vi "ReversedEngineering AnalyseStateMachineWhileLoop.vi"(0 "OutSideWhileLoop":refnum<vi>, 1 "StateWhileLoop":refnum<vi>, 2 "SelStrings":string[](array[string]), 5 "error in":errorcluster) -> (15 "InitialState":string, 16 "FinallState":string, 19 "error out":errorcluster)   [LabVIEW 2020]
panel:
  out "Array":string[](array[string])
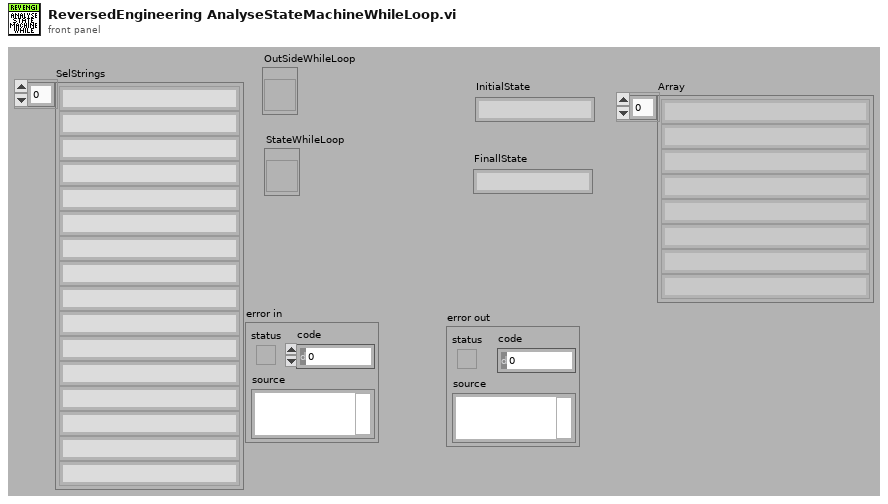
[diagram p1: front panel]
types:
  T1 = typedef "LVPositionTypeDef.ctl" = cluster{"Left":i32, "Top":i32}
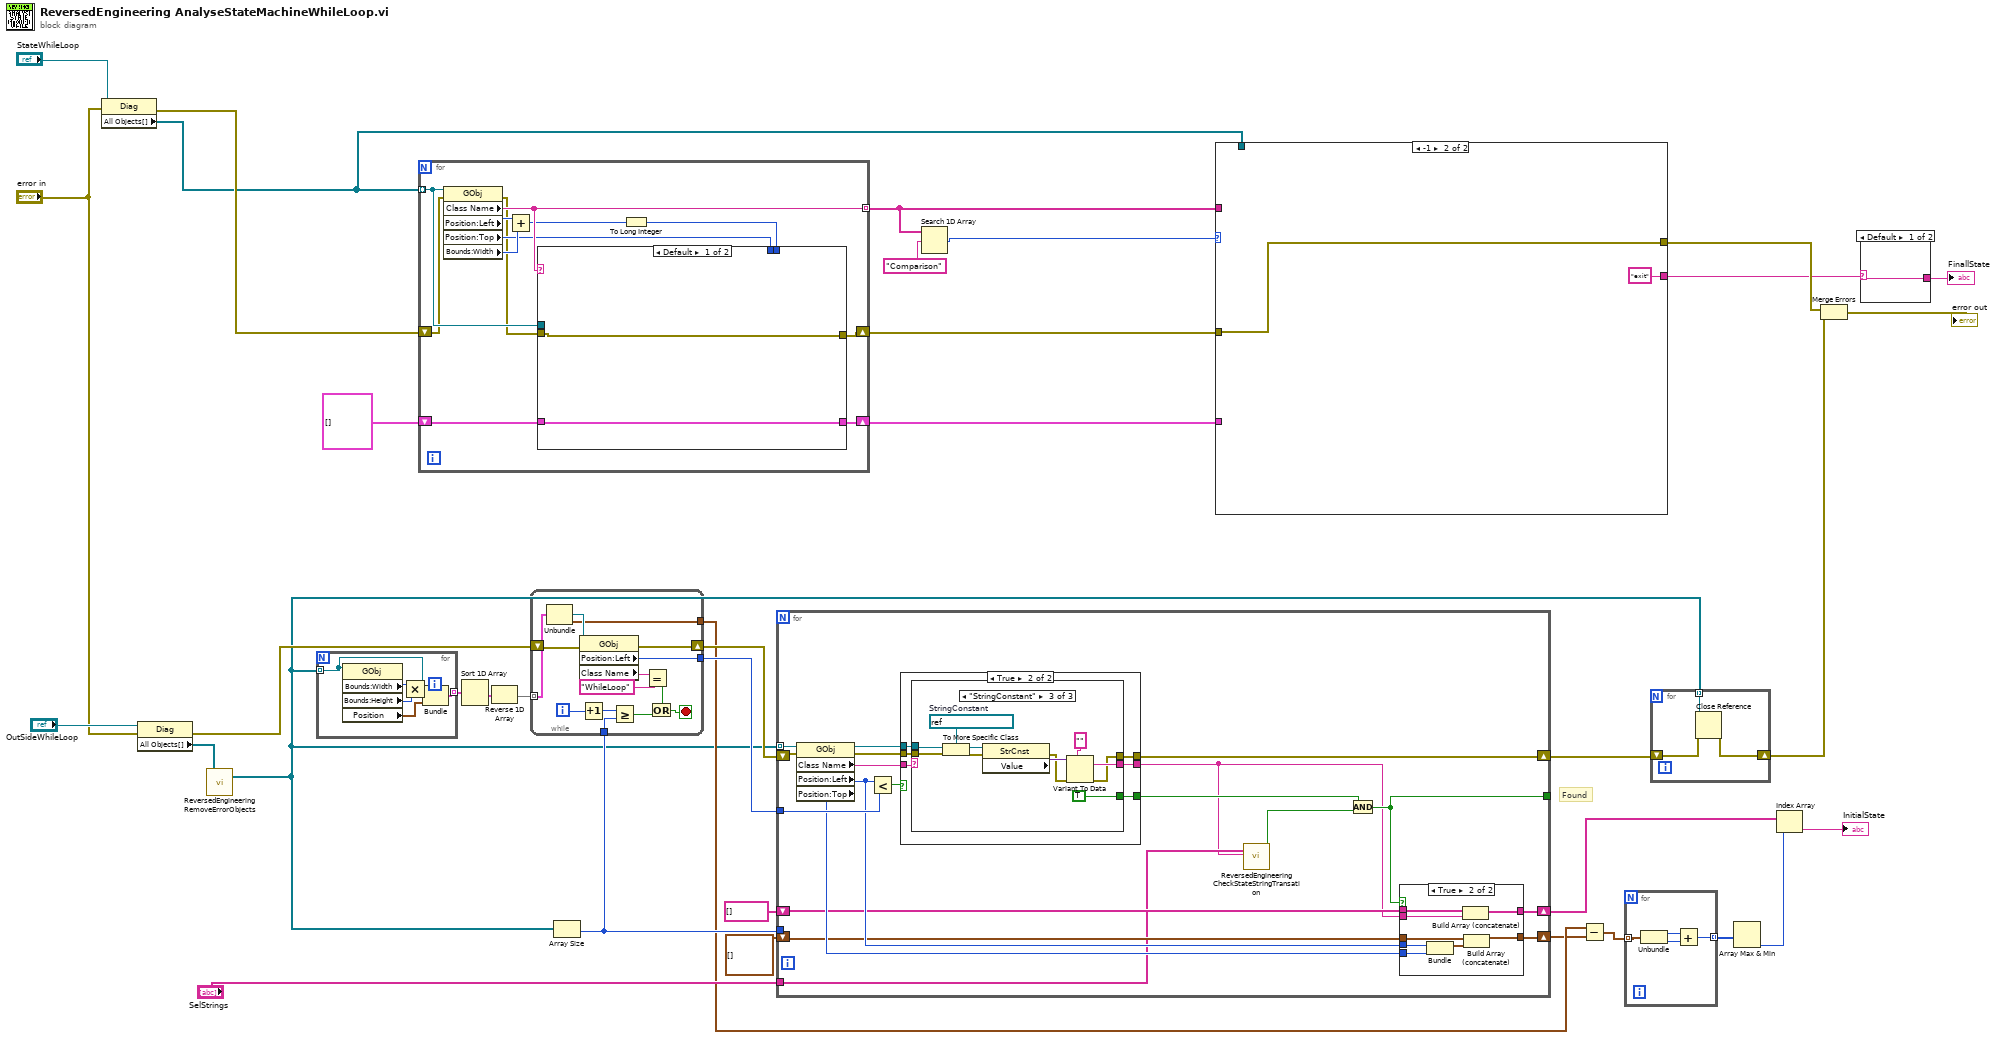
[diagram p0: block diagram]
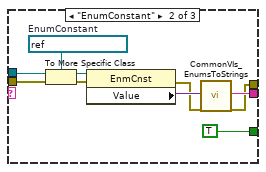
[diagram p5: hidden frame]
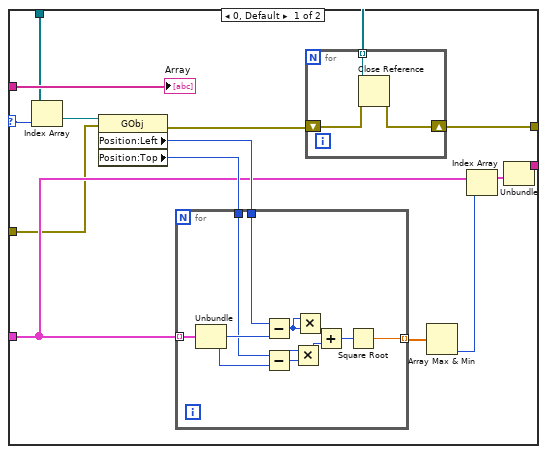
[diagram p6: hidden frame]
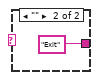
[diagram p7: hidden frame]
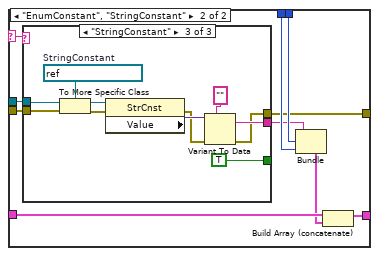
[diagram p8: hidden frame]
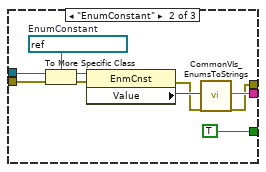
[diagram p10: hidden frame]
diagram:
  # "Found"
  n1 = property class="Diag"(reference="StateWhileLoop", error in="error in") -> (error out=w24:errorcluster, "All Objects[]"=w21:refnum<vi>[])  [unwired: 1 out]
  n2 = property class="Diag"(reference="OutSideWhileLoop", error in="error in") -> (error out=w31:errorcluster, "All Objects[]"=w2:refnum<vi>[])  [unwired: 1 out]
  n3 = call <resource>:"ReversedEngineering RemoveErrorObjects.vi"("ObjectsIn"=w2) -> ("ObjectsOut"=w1:refnum<vi>[])
  n4 = for {
    tunnel: w1 -> [w40] mode=indexing
    tunnel: [w41] -> w15 mode=indexing
    n5 = property class="GObj"(reference=w40) -> ("Bounds:Width"=w39:u32, "Bounds:Height"=w38:u32, "Position"=w37:T1)  [unwired: 1 in, 2 out]
    n6 = Multiply(x=w39, y=w38) -> (x*y=w42:u32)
    n7 = Bundle(w42, w40, "Position"=w37) -> (w41:cluster{u32, refnum<vi>, "Position":T1})  [unwired: 1 out]
  }
  n8 = for {
    tunnel: w21 -> [w49] mode=indexing
    tunnel: [w52] -> w28 mode=indexing
    shift-right: [w50] -> w25
    shift-left: cluster{"EnumItem":string, i32, "Top":i32}[] [] -> [w51]
    shift-right: [w44] -> w23
    shift-left: w24 -> [w45]
    n9 = property class="GObj"(reference=w49, error in=w45) -> (error out=w46:errorcluster, "Class Name"=w52:string, "Position:Left"=w54:i32, "Position:Top"=w47:i32, "Bounds:Width"=w53:u32)  [unwired: 1 out]
    n10 = Add(x=w54, y=w53) -> (x+y=w48:u32)
    n11 = To Long Integer(number=w48) -> (32bit integer=w43:i32)
    n12 = case shown="Default" w52 {
      selector: w52 -> [_ w62]
      tunnel: w51 -> [w55 w66]
      tunnel: [w55 w65] -> w50
      tunnel: w49 -> [_ w63]
      tunnel: w43 -> [_ w61]
      tunnel: w47 -> [_ w60]
      tunnel: w46 -> [w56 w59]
      tunnel: [w56 w57] -> w44
      frame Default {
      }
      frame "EnumConstant", "StringConstant" {
        n13 = case shown="\"StringConstant\"" w62 {
          tunnel: w63 -> [_ w77 w88]
          tunnel: [_ w73 w82] -> w58
          tunnel: [_ TRUE TRUE] -> _
          tunnel: w59 -> [w67 w71 w78]
          tunnel: [w67 w68 w81] -> w57
          frame "False", Default {
          }
          frame "EnumConstant" {
            w76 = refnum<vi> refnum  # EnumConstant
            n14 = To More Specific Class(target class=w76, reference=w77, error in=w71) -> (specific class reference=w75:refnum<vi>, error out=w70:errorcluster)
            n15 = property class="EnmCnst"(reference=w75, error in=w70) -> (error out=w69:errorcluster, "Value"=w74:variant)  [unwired: 1 out]
            n16 = call <resource>:"CommonVIs_EnumsToStrings.vi"("SingleEnumVariantIn"=w74, "error in (no error)"=w69) -> ("EnumItem"=w73:string, "error out"=w68:errorcluster)  [unwired: 1 in, 15 out]
          }
          frame "StringConstant" {
            w87 = refnum<vi> refnum  # StringConstant
            n17 = To More Specific Class(target class=w87, reference=w88, error in=w78) -> (specific class reference=w86:refnum<vi>, error out=w79:errorcluster)
            n18 = property class="StrCnst"(reference=w86, error in=w79) -> (error out=w80:errorcluster, "Value"=w84:variant)  [unwired: 1 out]
            n19 = Variant To Data(error in=w80, type="" ("EnumItem"), Variant=w84) -> (data=w82:string, error out=w81:errorcluster)
          }
        }
        n20 = Bundle("EnumItem"=w58, w61, "Top"=w60) -> (w64:cluster{"EnumItem":string, i32, "Top":i32})  [unwired: 1 out]
        n21 = Build Array (concatenate)(w66, w64) -> (w65:cluster{"EnumItem":string, i32, "Top":i32}[])
      }
    }
  }
  n22 = Sort 1D Array(array=w15) -> (sorted array=w14:cluster{u32, refnum<vi>, "Position":T1}[])
  n23 = Reverse 1D Array(array=w14) -> (reversed array=w13:cluster{u32, refnum<vi>, "Position":T1}[])
  n24 = Array Size(array=w1) -> (size(s)=w34:i32)
  n25 = while {
    tunnel: w13 -> [w91] mode=indexing
    tunnel: w34 -> [w101]
    tunnel: [w94] -> w33
    shift-right: [w93] -> w32
    shift-left: w31 -> [w92]
    tunnel: [w89] -> w4
    i -> [w100]
    stop <- w98 stop-if-true
    n26 = Unbundle(w91) -> (w90:refnum<vi>, "Position"=w89:T1)  [unwired: 1 out]
    n27 = property class="GObj"(reference=w90, error in=w92) -> (error out=w93:errorcluster, "Position:Left"=w94:i32, "Class Name"=w96:string)  [unwired: 1 out]
    n28 = Increment(x=w100) -> (x+1=w102:i32)
    n29 = Greater Or Equal?(x=w102, y=w101) -> (x >= y?=w99:bool)
    n30 = Equal?(x=w96, y="WhileLoop") -> (x = y?=w97:bool)
    n31 = Or(x=w97, y=w99) -> (x .or. y?=w98:bool)
  }
  n32 = for {
    tunnel: w1 -> [w119] mode=indexing
    tunnel: [w107] -> _
    tunnel: w34 -> [_]
    tunnel: w33 -> [w117]
    shift-right: [w114] -> w20
    shift-left: w32 -> [w116]
    shift-right: [w108] -> w8
    shift-left: string[] [] -> [w109]
    shift-right: [w110] -> w3
    shift-left: cluster{"Left":i32, "Top":i32}[] [] -> [w111]
    tunnel: "SelStrings" -> [w105]
    n33 = property class="GObj"(reference=w119, error in=w116) -> (reference out=w120:refnum<vi>, error out=w115:errorcluster, "Class Name"=w121:string, "Position:Left"=w113:i32, "Position:Top"=w112:i32)
    n34 = Less?(x=w113, y=w117) -> (x < y?=w118:bool)
    n35 = case shown="True" w118 {
      tunnel: w121 -> [_ w138]
      tunnel: w120 -> [_ w137]
      tunnel: [_ w136] -> w106
      tunnel: [_ w135] -> w104
      tunnel: w115 -> [w132 w134]
      tunnel: [w132 w133] -> w114
      frame False {
      }
      frame True {
        n36 = case shown="\"StringConstant\"" w138 {
          tunnel: w137 -> [_ w149 w160]
          tunnel: [_ w145 w154] -> w135
          tunnel: [_ TRUE TRUE] -> w136
          tunnel: w134 -> [w139 w143 w150]
          tunnel: [w139 w140 w153] -> w133
          frame Default {
          }
          frame "EnumConstant" {
            w148 = refnum<vi> refnum  # EnumConstant
            n37 = To More Specific Class(target class=w148, reference=w149, error in=w143) -> (specific class reference=w147:refnum<vi>, error out=w142:errorcluster)
            n38 = property class="EnmCnst"(reference=w147, error in=w142) -> (error out=w141:errorcluster, "Value"=w146:variant)  [unwired: 1 out]
            n39 = call <resource>:"CommonVIs_EnumsToStrings.vi"("SingleEnumVariantIn"=w146, "error in (no error)"=w141) -> ("EnumItem"=w145:string, "error out"=w140:errorcluster)  [unwired: 1 in, 15 out]
          }
          frame "StringConstant" {
            w159 = refnum<vi> refnum  # StringConstant
            n40 = To More Specific Class(target class=w159, reference=w160, error in=w150) -> (specific class reference=w158:refnum<vi>, error out=w151:errorcluster)
            n41 = property class="StrCnst"(reference=w158, error in=w151) -> (error out=w152:errorcluster, "Value"=w156:variant)  [unwired: 1 out]
            n42 = Variant To Data(error in=w152, type="" ("EnumItem"), Variant=w156) -> (data=w154:string, error out=w153:errorcluster)
          }
        }
      }
    }
    n43 = call <resource>:"ReversedEngineering CheckStateStringTransation.vi"("SelStrings"=w105, "StringConstant"=w104) -> ("Found"=w103:bool)  [unwired: 2 in, 15 out]
    n44 = And(x=w106, y=w103) -> (x .and. y?=w107:bool)
    n45 = case shown="True" w107 {
      tunnel: w113 -> [_ w131]
      tunnel: w112 -> [_ w130]
      tunnel: w111 -> [w123 w128]
      tunnel: [w123 w127] -> w110
      tunnel: w109 -> [w122 w126]
      tunnel: [w122 w125] -> w108
      tunnel: w104 -> [_ w124]
      frame False {
      }
      frame True {
        n46 = Bundle("Left"=w131, "Top"=w130) -> (w129:cluster{"Left":i32, "Top":i32})  [unwired: 1 out]
        n47 = Build Array (concatenate)(w126, w124) -> (w125:string[])
        n48 = Build Array (concatenate)(w128, w129) -> (w127:cluster{"Left":i32, "Top":i32}[])
      }
    }
  }
  n49 = Search 1D Array(1D array=w28, element="Comparison") -> (index of element=w16:i32)  [unwired: 1 out]
  n50 = case shown="-1" w16 {
    selector: w16 -> [w161 _]
    tunnel: w28 -> [w174 _]
    tunnel: w25 -> [w169 _]
    tunnel: w23 -> [w166 w190]
    tunnel: [w164 w190] -> w22
    tunnel: w21 -> [w163 _]
    tunnel: [w162 "exit" ("EnumItem")] -> w18
    frame 0, Default {
      n51 = Index Array(array=w163, index=w161) -> (element=w173:refnum<vi>)
      n52 = property class="GObj"(reference=w173, error in=w166) -> (error out=w165:errorcluster, "Position:Left"=w172:i32, "Position:Top"=w171:i32)  [unwired: 1 out]
      n53 = for {
        tunnel: w169 -> [w188] mode=indexing
        tunnel: w172 -> [w187]
        tunnel: w171 -> [w185]
        tunnel: [w178] -> w170 mode=indexing
        n54 = Unbundle(w188) -> (w186:i32, "Top"=w184:i32)  [unwired: 1 out]
        n55 = Subtract(x=w187, y=w186) -> (x-y=w183:i32)
        n56 = Subtract(x=w185, y=w184) -> (x-y=w182:i32)
        n57 = Multiply(x=w182, y=w182) -> (x*y=w180:i32)
        n58 = Multiply(x=w183, y=w183) -> (x*y=w181:i32)
        n59 = Add(x=w181, y=w180) -> (x+y=w179:i32)
        n60 = Square Root(x=w179) -> (sqrt(x)=w178:dbl)
      }
      n61 = for {
        shift-right: [w176] -> w164
        shift-left: w165 -> [w177]
        tunnel: w163 -> [w175] mode=indexing
        n62 = Close Reference(reference=w175, error in (no error)=w177) -> (error out=w176:errorcluster)
      }
      n63 = Array Max & Min(array=w170) -> (min index (indices)=w168:i32)  [unwired: 3 out]
      n64 = Index Array(array=w169, index=w168) -> (element=w167:cluster{"EnumItem":string, i32, "Top":i32})
      n65 = Unbundle(w167) -> ("EnumItem"=w162:string)  [unwired: 2 out]
      "Array" <- w174
    }
    frame -1 {
    }
  }
  n66 = Subtract(x=w4, y=w3) -> (x-y=w11:T1[])
  n67 = for {
    tunnel: w11 -> [w194] mode=indexing
    tunnel: [w191] -> w10 mode=indexing
    n68 = Unbundle(w194) -> ("Left"=w193:i32, "Top"=w192:i32)
    n69 = Add(x=w193, y=w192) -> (x+y=w191:i32)
  }
  n70 = for {
    shift-right: [w196] -> w19
    shift-left: w20 -> [w197]
    tunnel: w1 -> [w195] mode=indexing
    n71 = Close Reference(reference=w195, error in (no error)=w197) -> (error out=w196:errorcluster)
  }
  n72 = Array Max & Min(array=w10) -> (min index (indices)=w9:i32)  [unwired: 3 out]
  n73 = Index Array(array=w8, index=w9) -> (element=→"InitialState":string)
  n74 = Merge Errors(w22, w19) -> (→"error out":errorcluster)
  n75 = case shown="Default" w18 {
    selector: w18 -> [w198 _]
    tunnel: [w198 "Exit" ("FinallState")] -> w17
    frame Default {
    }
    frame "" {
    }
  }
  "FinallState" <- w17
